vi "Mark Items as Expired.vi"(10 "Expired Tags":string[](array[string]), 11 "Process Tree View Model in":refnum<class "Process Tree View Model.lvclass">) -> (3 "Process Tree View Model out":refnum<class "Process Tree View Model.lvclass">)   [LabVIEW 2020, in "Process Tree View Model.lvclass"]
uses:
  Process Tree View Model.lvclass
  Process Tree View Model.lvclass/Process Tree View Model.ctl
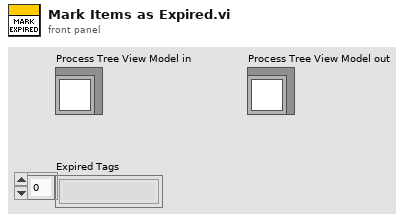
[diagram p1: front panel]
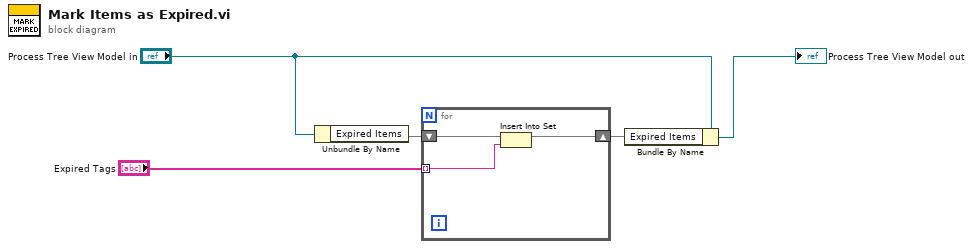
[diagram p0: block diagram]
diagram:
  n1 = Unbundle By Name("Process Tree View Model in") -> ("Expired Items"=w1:set{string})
  n2 = for {
    shift-right: [w7] -> w4
    shift-left: w1 -> [w8]
    tunnel: "Expired Tags" -> [w6] mode=indexing
    n3 = Insert Into Set(10:w6, 11:w8) -> (3:w7:set{string})  [unwired: 1 out]
  }
  n4 = Bundle By Name(cluster="Process Tree View Model in", "Expired Items"=w4) -> (→"Process Tree View Model out":refnum<class "Process Tree View Model.lvclass">)
